vi "Stop Scan Core.vi"(8 "error in (no error)":errorcluster, 11 "CS++MCS in":refnum<class "CS++MCS.lvclass">) -> (0 "error out":errorcluster, 3 "CS++MCS out":refnum<class "CS++MCS.lvclass">)   [LabVIEW 2015, in "CS++MCS.lvlib" / "CS++MCS.lvclass"]
doc: "This VI stops a scan."
uses:
  CS++MCS.lvclass
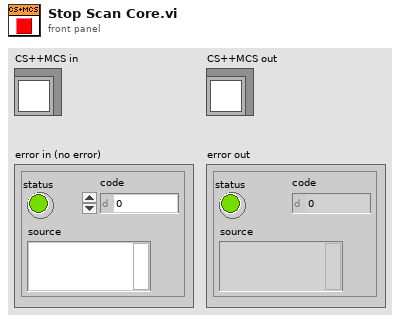
[diagram p1: front panel]
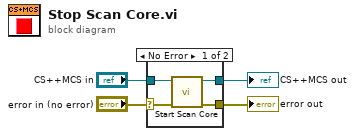
[diagram p0: block diagram]
diagram:
  n1 = case shown="No Error" "error in (no error)" {
    selector: "error in (no error)" -> [w6 w10]
    tunnel: [w5 w10] -> w3
    tunnel: [w7 w9] -> w1
    tunnel: "CS++MCS in" -> [w8 w9]
    frame No Error {
      n2 = call-dynamic "Start Scan Core.vi"("error in (no error)"=w6, "CS++MCS in"=w8) -> ("error out"=w5:errorcluster, "CS++MCS out"=w7:refnum<class "CS++MCS.lvclass">)  [unwired: 8 in]
    }
    frame Error {
    }
  }
  "error out" <- w3
  "CS++MCS out" <- w1
